vi "swag 3.vi"(1 "°Farenheit":dbl) -> (0 "Rankine":dbl(slide) scale=-100.0..1000.0)   [LabVIEW 2014]
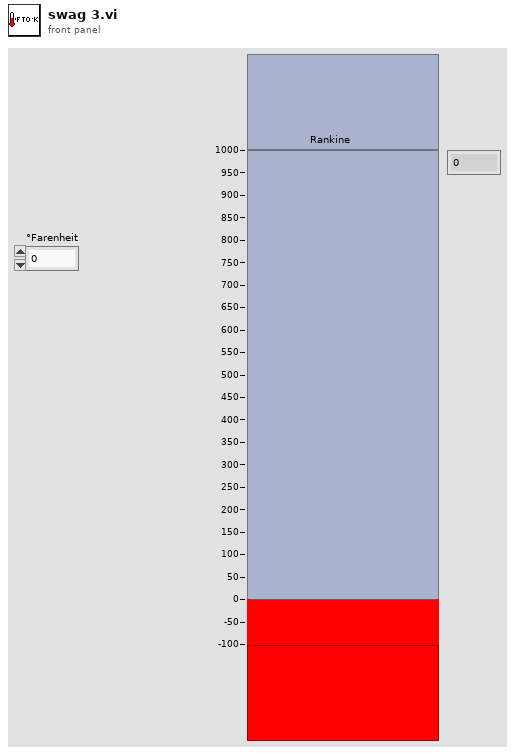
[diagram p1: front panel]
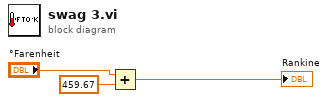
[diagram p0: block diagram]
diagram:
  n1 = Add(x="°Farenheit", y=459.67) -> (x+y=→"Rankine":dbl)
